vi "VI Build.vi"   [LabVIEW 2020]
uses:
  <vilib>/AppBuilder/AB_API_Simple/Build (path).vi
  <vilib>/AppBuilder/AB_API_Simple/NI_App_Builder_API.lvlib
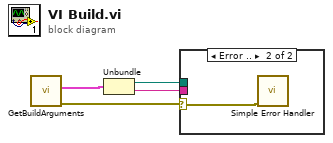
[diagram p0: block diagram]
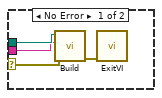
[diagram p2: hidden frame]
diagram:
  n1 = call "GetBuildArguments.vi"() -> ("error out"=w1:errorcluster, "output cluster"=w4:cluster{"Path ":path, string})  [unwired: 10 in]
  n2 = Unbundle(w4) -> ("Path"=w3:path, w2:string)
  n3 = case shown="Error .." w1 {
    selector: w1 -> [w5 w9]
    tunnel: w3 -> [w7 _]
    tunnel: w2 -> [w6 _]
    frame No Error {
      n4 = call-poly <vilib>:"Build.vi"("error in (no error)"=w5, "Name of build specification (if empty: build all)"=w6, "Path to project"=w7) -> ("error out"=w8:errorcluster)  [unwired: 7 in, 1 out]
      n5 = call "ExitVI.vi"("error in (no error)"=w8) -> ()  [unwired: 10 in, 1 out]
    }
    frame Error {
      n6 = call <vilib>:"Simple Error Handler.vi"("error in (no error)"=w9) -> ()  [unwired: 4 in, 5 out]
    }
  }
